vi "DAQ.vi"() -> (1 "Rt":dbl format="%0.2f", 2 "LM35":dbl format="%0.2f")   [LabVIEW 2020]
uses:
  <vilib>/Analysis/baseanly.llb/Mean (DBL).vi
  <vilib>/Analysis/NI_AALBase.lvlib
panel:
  out "波形图表":dynamicdata(graph)
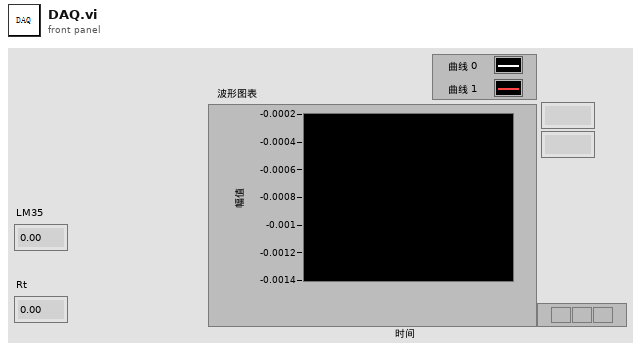
[diagram p1: front panel]
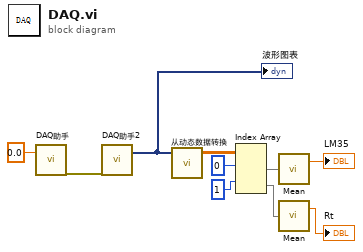
[diagram p0: block diagram]
diagram:
  n1 = call "DAQ助手"("data"=0.0 ("数据")) -> ("error out"=w10:errorcluster)  [unwired: 17 in, 1 out]
  n2 = call "DAQ助手2"("error in"=w10) -> ("data"=w1:dynamicdata)  [unwired: 16 in, 2 out]
  "波形图表" <- w1
  n3 = call "从动态数据转换"("Dynamic Data Type"=w1) -> ("Array"=w7:dbl[][])  [unwired: 3 in]
  n4 = Index Array(array=w7, index (row) #1=0 ("索引"), index (row) #2=1 ("索引 (行)")) -> (element #1=w5:dbl[], element #2=w4:dbl[])  [unwired: 2 in]
  n5 = call-poly <vilib>:"Mean.vi"("X"=w5) -> ("mean"=→"LM35":dbl)  [unwired: 1 out]
  n6 = call-poly <vilib>:"Mean.vi"("X"=w4) -> ("mean"=→"Rt":dbl)  [unwired: 1 out]
